vi "joystik 1.vi"() -> ()   [LabVIEW 2019]
uses:
  <vilib>/Utility/inputDevices.llb/joystickAcquire.vi
  <vilib>/Utility/inputDevices.llb/closeJoystick.vi
panel:
  out "error out":errorcluster
  in  "stop":bool
  out "axis info":T1
  out "button info":T2
  out "direction info":T3
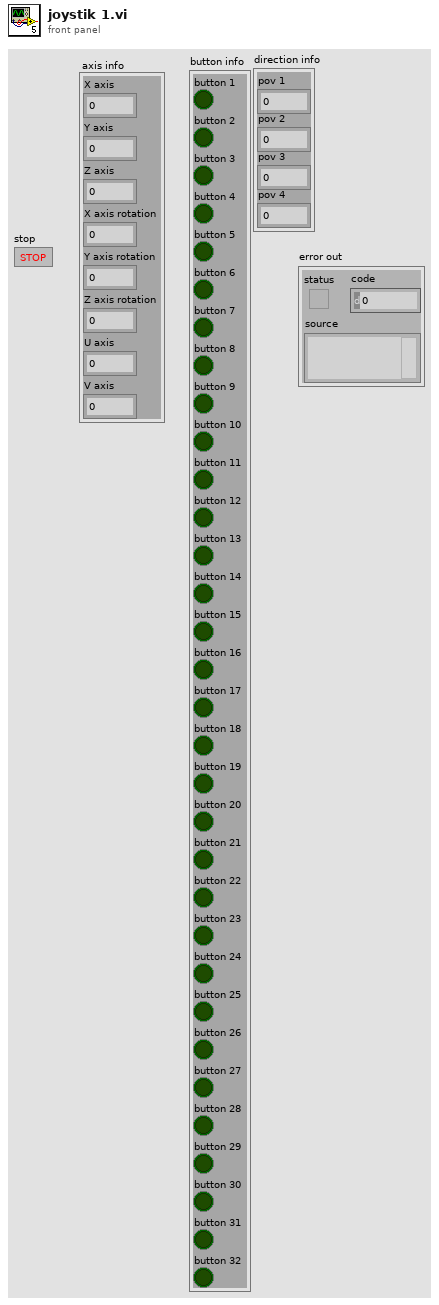
[diagram p1: front panel]
types:
  T1 = cluster{"X axis":i32, "Y axis":i32, "Z axis":i32, "X axis rotation":i32, "Y axis rotation":i32, "Z axis rotation":i32, "U axis":i32, "V axis":i32}
  T2 = cluster{"button 1":bool, "button 2":bool, "button 3":bool, "button 4":bool, "button 5":bool, "button 6":bool, "button 7":bool, "button 8":bool, "button 9":bool, "button 10":bool, "button 11":bool, "button 12":bool, "button 13":bool, "button 14":bool, "button 15":bool, "button 16":bool, "button 17":bool, "button 18":bool, "button 19":bool, "button 20":bool, "button 21":bool, "button 22":bool, "button 23":bool, "button 24":bool, "button 25":bool, "button 26":bool, "button 27":bool, "button 28":bool, "button 29":bool, "button 30":bool, "button 31":bool, "button 32":bool}
  T3 = cluster{"pov 1":i32, "pov 2":i32, "pov 3":i32, "pov 4":i32}
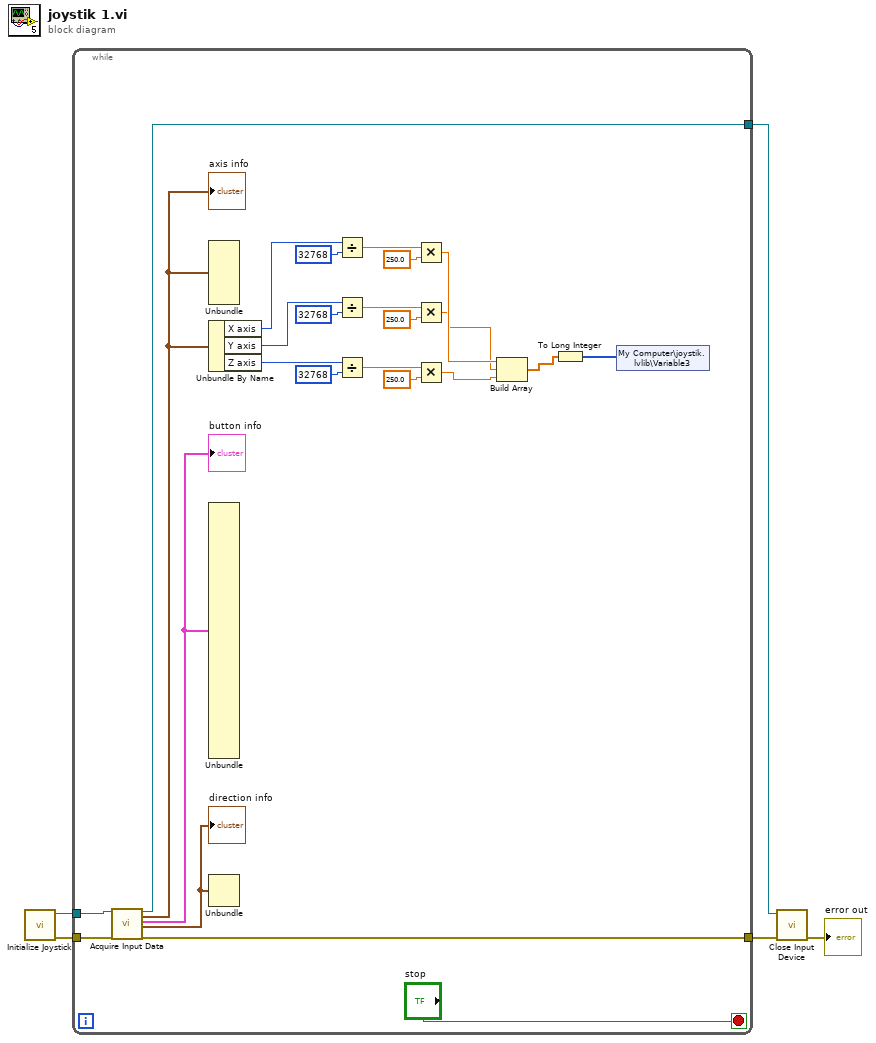
[diagram p0: block diagram]
diagram:
  n1 = call <vilib>:"Initialize Joystick.vi"() -> ("error out"=w4:errorcluster, "device ID"=w5:refnum<k1>)  [unwired: 10 in]
  n2 = while {
    tunnel: w5 -> [w29]
    tunnel: w4 -> [w28]
    tunnel: [w27] -> w3
    tunnel: [w26] -> w2
    stop <- "stop" stop-if-true
    n3 = call-poly <vilib>:"Acquire Input Data.vi"("device ID"=w29, "error in (no error)"=w28) -> ("device ID"=w26:refnum<k1>, "axis info"=w23:T1, "button info"=w25:T2, "direction info"=w24:T3, "error out"=w27:errorcluster)  [unwired: 13 in]
    "axis info" <- w23
    "button info" <- w25
    "direction info" <- w24
    n4 = Unbundle(w23) -> ()  [unwired: 8 out]
    n5 = Unbundle By Name(w23) -> ("X axis"=w22:i32, "Y axis"=w21:i32, "Z axis"=w20:i32)
    n6 = Unbundle(w25) -> ()  [unwired: 32 out]
    n7 = Unbundle(w24) -> ()  [unwired: 4 out]
    n8 = Divide(x=w22, y=32768) -> (x/y=w16:dbl)
    n9 = Divide(x=w21, y=32768) -> (x/y=w14:dbl)
    n10 = Divide(x=w20, y=32768) -> (x/y=w12:dbl)
    n11 = Multiply(x=w16, y=250.0) -> (x*y=w10:dbl)
    n12 = Multiply(x=w14, y=250.0) -> (x*y=w9:dbl)
    n13 = Multiply(x=w12, y=250.0) -> (x*y=w8:dbl)
    n14 = Build Array(w10, w9, w8) -> (w7:dbl[])
    n15 = To Long Integer(number=w7) -> (32bit integer=w6:i32[])
    n16 = shared-variable "My Computer\\joystik.lvlib\\Variable3"(w6) -> ()  [unwired: 1 in, 1 out]
  }
  n17 = call-poly <vilib>:"Close Input Device.vi"("error in (no error)"=w3, "device ID"=w2) -> ("error out"=→"error out":errorcluster)  [unwired: 8 in]
